vi "Format position command.vi"(9 "Zcommand (steps)":dbl format="%.4f", 10 "Ycommand (steps)":dbl format="%.4f", 11 "Xcommand (steps)":dbl format="%.4f") -> (3 "concatenated string":string)   [LabVIEW 2010]
panel:
  out "unsigned byte array":u8[](array[numeric])
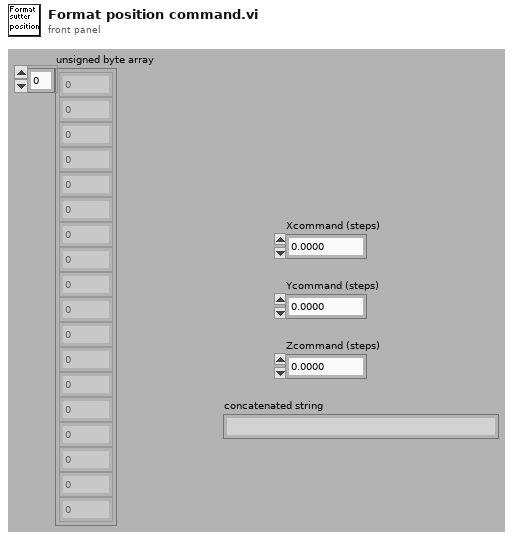
[diagram p1: front panel]
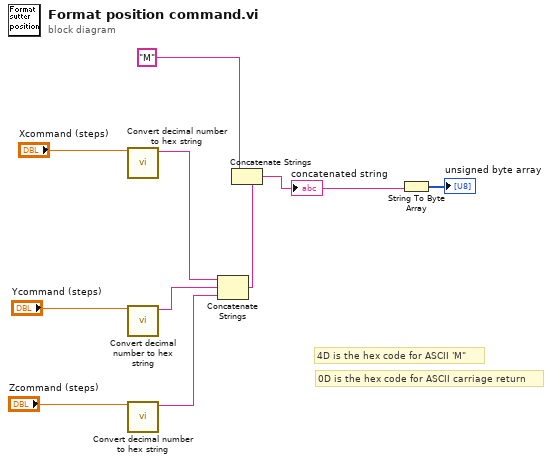
[diagram p0: block diagram]
diagram:
  # "0D is the hex code for ASCII carriage return"
  # "4D is the hex code for ASCII 'M\""
  n1 = call "Convert decimal number to hex string.vi"("Decimal number"="Xcommand (steps)") -> ("Hexadecimal command string"=w4:string)  [unwired: 10 out]
  n2 = call "Convert decimal number to hex string.vi"("Decimal number"="Ycommand (steps)") -> ("Hexadecimal command string"=w3:string)  [unwired: 10 out]
  n3 = call "Convert decimal number to hex string.vi"("Decimal number"="Zcommand (steps)") -> ("Hexadecimal command string"=w2:string)  [unwired: 10 out]
  n4 = Concatenate Strings(w4, w3, w2) -> (w1:string)
  n5 = Concatenate Strings("M" ("Hexadecimal command string"), w1) -> (w6:string)
  "concatenated string" <- w6
  n6 = String To Byte Array(string=w6) -> (unsigned byte array=→"unsigned byte array":u8[])
